vi "2013_01_05 Durability8 debug.vi"() -> ()   [LabVIEW 2012]
uses:
  MotorTypeDef.ctl
  <vilib>/DAQmx/write.llb/DAQmx Write (Counter Time 1Chan 1Samp).vi
  <vilib>/DAQmx/read.llb/DAQmx Read (Analog 1D Wfm NChan NSamp).vi
  <vilib>/Utility/TradDaqScaling.llb/Convert Thermistor Reading (waveform).vi
  <vilib>/DAQmx/miscellaneous.llb/DAQmx Fill In Error Info.vi
panel:
  out "XY Graph 2":cluster{"Array":dbl[], "Array":dbl[]}[](graph)
  out "Single Motor 2":waveform(dbl)[](graph)
  in  "Waveform":bool
  in  "Motor":dbl=1.0 min=1.0 max=8.0 step=1.0
  out "XY Graph":cluster{"Array":dbl[], "Array":dbl[]}(graph)
  out "error out":errorcluster
  in  "File Path":path=path "Durability/.lvm"
  in  "Motor 1":T1 {"Power Input (W)" format="%.3g"; "Efficiency" format="%#_3g%%"; "Power Output (W)" format="%.3g"; "Torque (mNm)" format="%.3g"; "Elapsed Time" format="%<%H:%M:%S>t"; "Supply (V)" format="%.2f"; "RPM" scale=0.0..40000.0 scale format="%#_4p"}
  out "Motor Temp":dbl(slide) scale=65.0..110.0
  out "Tank Temp":dbl(slide) scale=65.0..110.0
  in  "Temp Probe\nOn Motor":dbl=1.0
  out "loop time (ms)":u32
  in  "stop":bool
  in  "Unlock PWM":bool=TRUE
  in  "PWM 2":dbl(slide)=100.0 min=0.0 max=100.0 step=5.0 scale=0.0..100.0
  in  "PWM 1":dbl(slide) min=0.0 max=100.0 step=5.0 scale=0.0..100.0
  # "Enable"
  # "Fail"
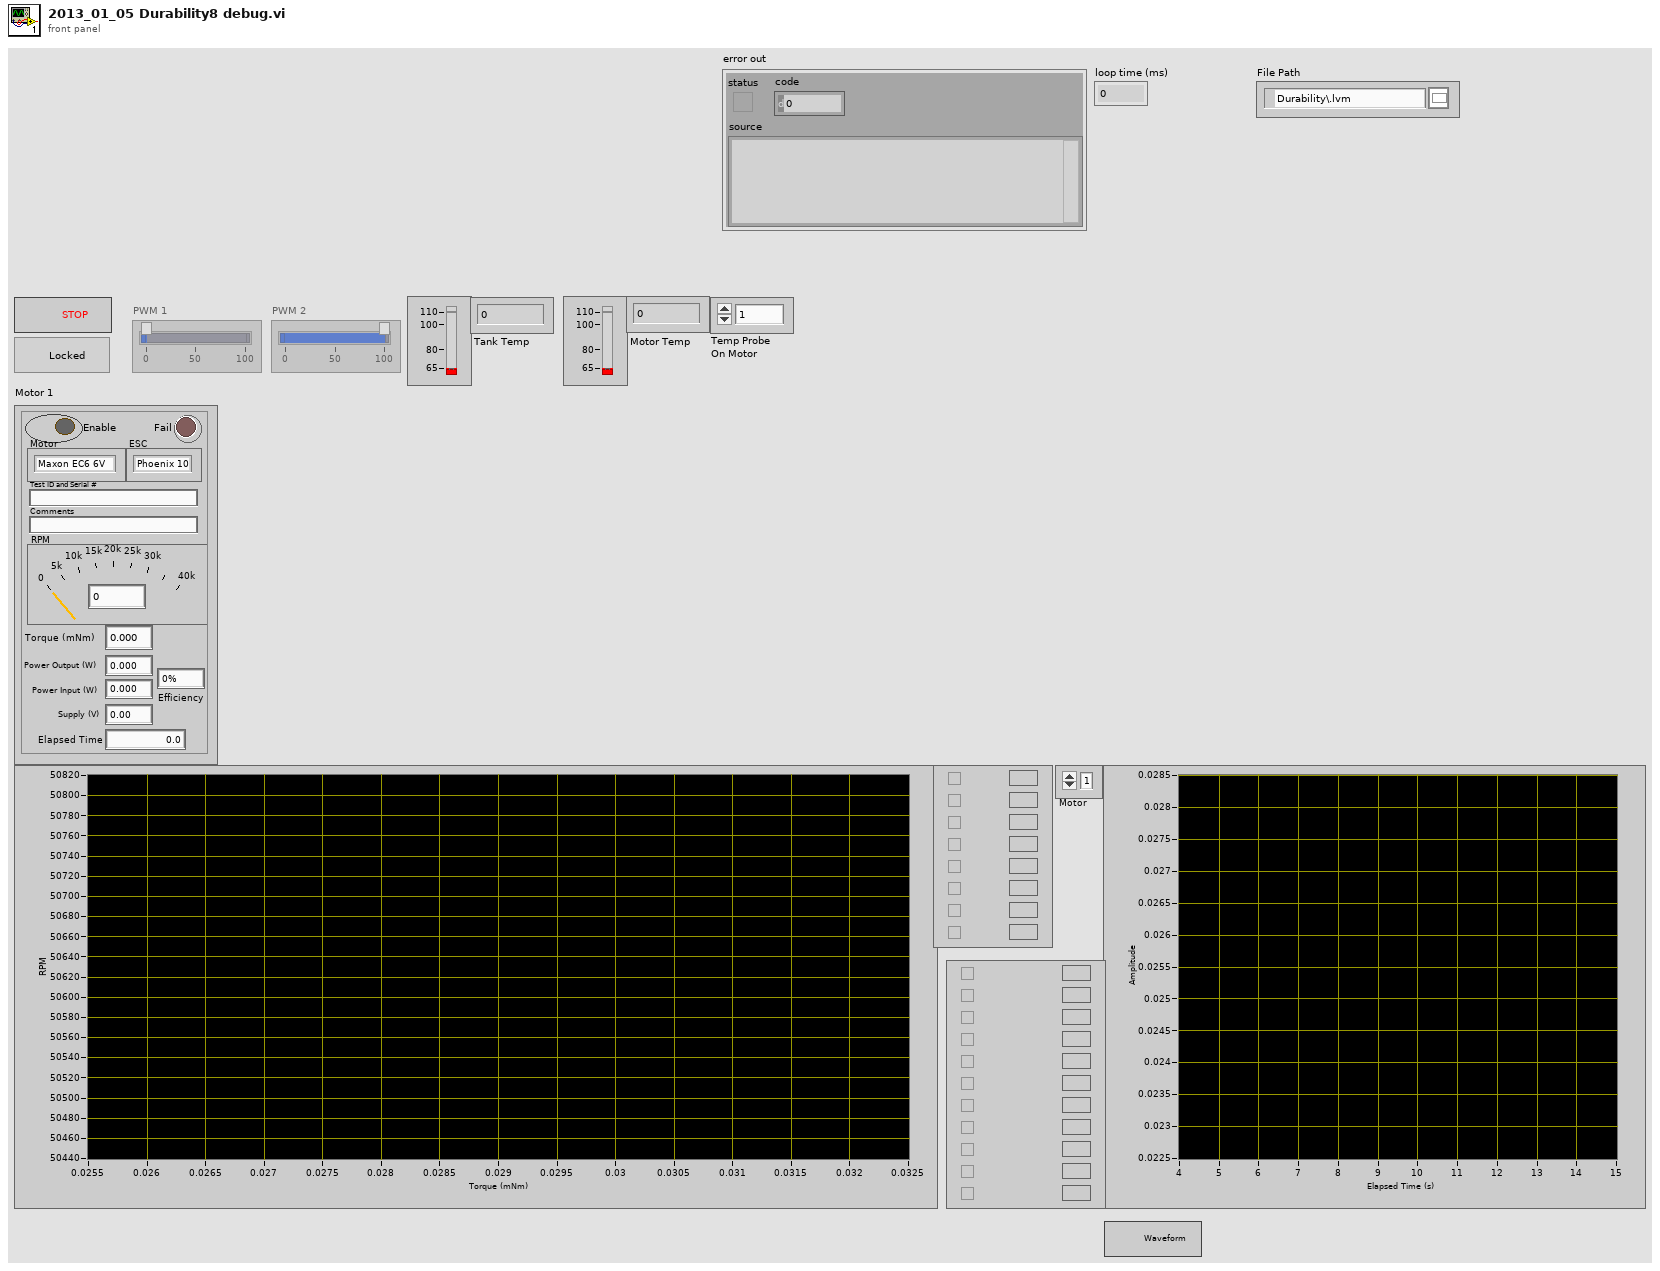
[diagram p1: front panel]
types:
  T1 = typedef "MotorTypeDef.ctl" = cluster{"Enabled":bool, "Fail":bool, "RPM":dbl, "Motor":enum16{"Maxon EC6 6V", "Maxon EC4 6V", "FH 0620 6V", "FH 0620 12V"}, "ESC":enum16{"Phoenix 10", "Maxon", "FH 1801"}, "Supply (V)":dbl, "Test ID and Serial #":string, "Comments":string, "Elapsed Time":dbl, "Counter":dbl, "Torque (mNm)":dbl, "Power Output (W)":dbl, "Efficiency":dbl, "Power Input (W)":dbl}
  T2 = enum8{"Enabled", "Disabled", "Disabled and Grayed Out"}
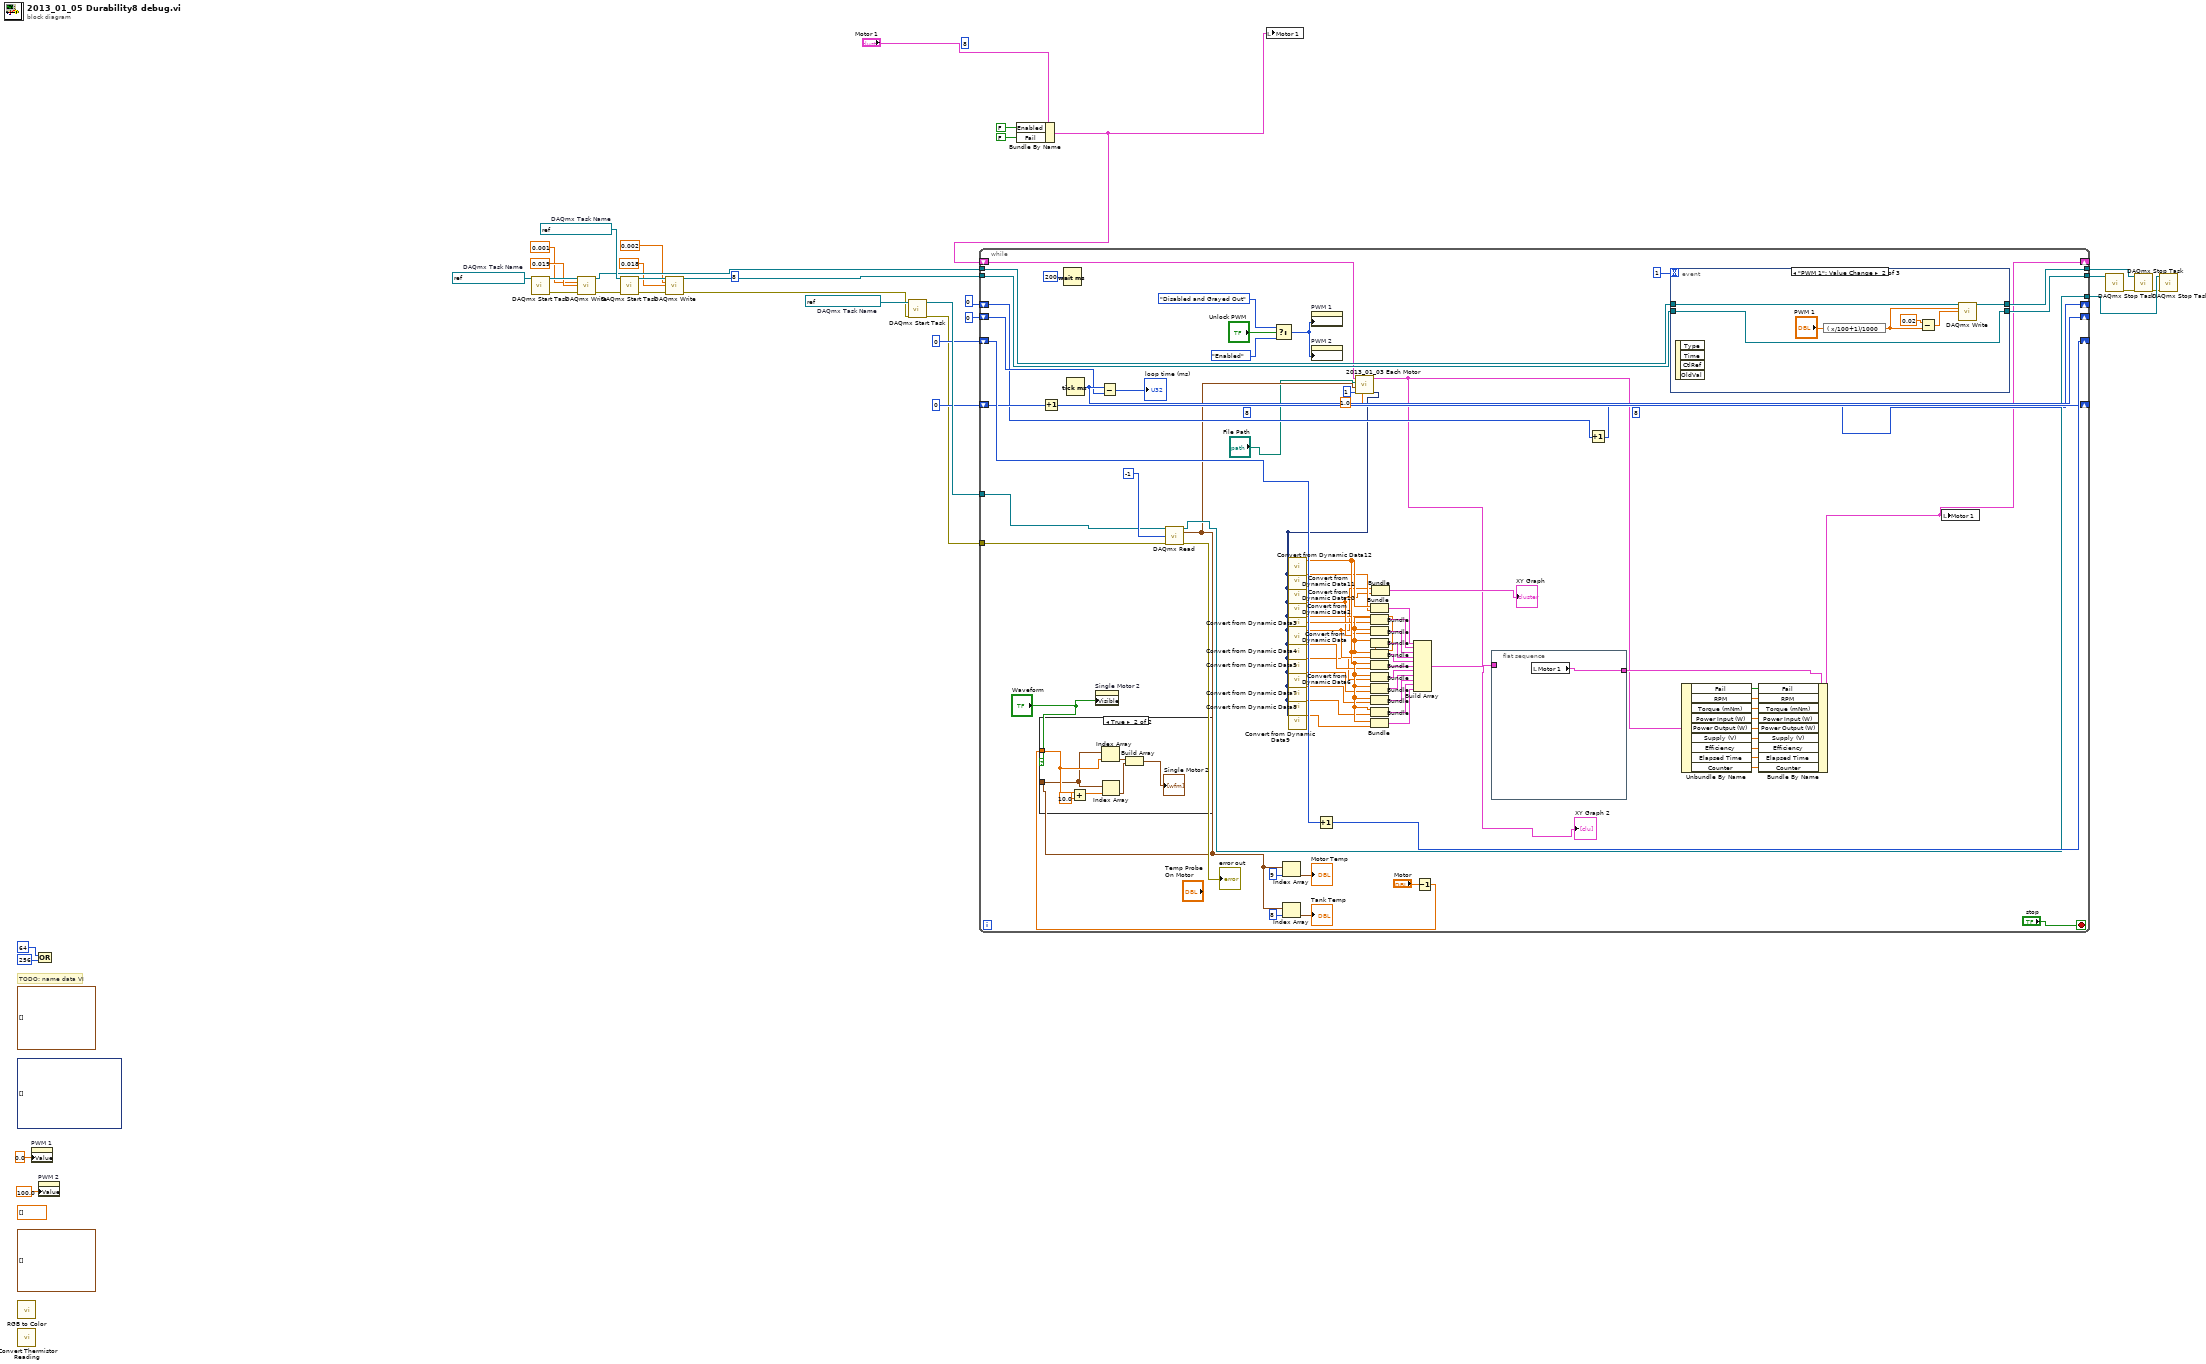
[diagram p0: block diagram]
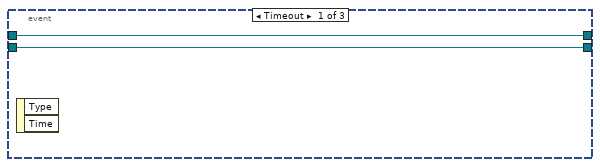
[diagram p3: hidden frame]
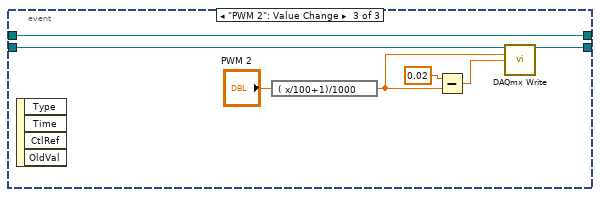
[diagram p4: hidden frame]
diagram:
  (unwired) 8
  (unwired) 8
  (unwired) dynamicdata[] []
  (unwired) dbl[] [] ("History Data")
  (unwired) waveform(dbl)[][] [] ("History Data")
  (unwired) waveform(dbl)[][] [] ("History Data")
  w30 = refnum<k21> "Durability8 PWM2"  # DAQmx Task Name
  w31 = refnum<k21> "Durability8 PWM1"  # DAQmx Task Name
  w34 = refnum<k21> "Durability8 Acquire"  # DAQmx Task Name
  # "TODO: name data VI"
  n1 = call <vilib>:"RGB to Color.vi"() -> ()  [unwired: 3 in, 1 out]
  n2 = call-poly <vilib>:"Convert Thermistor Reading.vi"() -> ()  [unwired: 7 in, 1 out]
  n3 = property on="PWM 1" class="Slide (strict)"("Value"=0.0 ("PWM 1")) -> ()  [unwired: 2 in, 2 out]
  n4 = Compound Arithmetic op=OR(64 ("options"), 256 ("options")) -> ()  [unwired: 1 out]
  n5 = property on="PWM 2" class="Slide (strict)"("Value"=100.0 ("PWM 2")) -> ()  [unwired: 2 in, 2 out]
  n6 = call <vilib>:"DAQmx Start Task.vi"("task/channels in"=w31) -> ("task out"=w27:refnum<k21>, "error out"=w25:errorcluster)  [unwired: 13 in]
  n7 = call-poly <vilib>:"DAQmx Write.vi"("task/channels in"=w27, "high time"=0.001 ("data"), "low time"=0.019 ("data"), "error in"=w25) -> ("task out"=w29:refnum<k21>, "error out"=w24:errorcluster)  [unwired: 9 in, 1 out]
  n8 = call <vilib>:"DAQmx Start Task.vi"("task/channels in"=w30, "error in"=w24) -> ("task out"=w26:refnum<k21>, "error out"=w23:errorcluster)  [unwired: 12 in]
  n9 = call-poly <vilib>:"DAQmx Write.vi"("task/channels in"=w26, "high time"=0.002 ("data"), "low time"=0.018 ("data"), "error in"=w23) -> ("task out"=w28:refnum<k21>, "error out"=w5:errorcluster)  [unwired: 9 in, 1 out]
  n10 = call <vilib>:"DAQmx Start Task.vi"("task/channels in"=w34, "error in"=w5) -> ("task out"=w33:refnum<k21>, "error out"=w6:errorcluster)  [unwired: 12 in]
  n11 = Bundle By Name(cluster="Motor 1", "Enabled"=FALSE, "Fail"=FALSE) -> (w1:T1)
  n12 = while {
    tunnel: w33 -> [w79]
    tunnel: [w80] -> w32
    tunnel: w6 -> [w92]
    shift-right: [w105] -> _
    shift-left: u32 0 ("millisecond timer value") -> [w104]
    tunnel: w29 -> [w97]
    tunnel: w28 -> [w96]
    tunnel: [w95] -> w22
    tunnel: [w94] -> w15
    shift-right: [w90] -> _
    shift-left: 0 ("for") -> [w91]
    shift-right: [w66] -> _
    shift-left: 0 ("for") -> [w67]
    shift-right: [w88] -> _
    shift-left: 0 ("for") -> [w89]
    shift-right: [w35] -> _
    shift-left: w1 -> [w78]
    stop <- "stop" stop-if-true
    (unwired) 8
    (unwired) 8
    n13 = Increment(x=w89) -> (x+1=w88:i32)
    n14 = Wait (ms)(milliseconds to wait=u32 200) -> ()  [unwired: 1 out]
    n15 = Tick Count (ms)() -> (millisecond timer value=w105:u32)
    n16 = property on="Single Motor 2" class="WFGraph (strict)"("Visible"="Waveform") -> ()  [unwired: 2 in, 2 out]
    n17 = Subtract(x=w105, y=w104) -> (x-y=→"loop time (ms)":u32)
    n18 = call-poly <vilib>:"DAQmx Read.vi"("task/channels in"=w79, "number of samples per channel"=-1, "error in"=w92) -> ("task out"=w80:refnum<k21>, "data"=w41:waveform(dbl)[], "error out"=→"error out":errorcluster)  [unwired: 10 in]
    n19 = Select(t=T2."Disabled and Grayed Out" ("Disabled"), s="Unlock PWM", f=T2."Enabled" ("Disabled")) -> (s? t:f=w109:T2)
    n20 = Index Array(array=w41, index=9) -> (element=→"Motor Temp":waveform(dbl))
    n21 = Index Array(array=w41, index=8) -> (element=→"Tank Temp":waveform(dbl))
    n22 = property on="PWM 1" class="Slide (strict)"("DisabledEnum"=w109) -> ()  [unwired: 2 in, 2 out]
    n23 = property on="PWM 2" class="Slide (strict)"("DisabledEnum"=w109) -> ()  [unwired: 2 in, 2 out]
    n24 = Increment(x=w91) -> (x+1=w90:i32)
    n25 = call "2013_01_03 Each Motor.vi"("Temp On"=1.0, "Motor #"=1, "data"=w41, "File Path"="File Path", "Motor Typedef"=w78) -> ("Final Out"=w38:dynamicdata, "Motor Typedef Out"=w36:T1)  [unwired: 5 in]
    n26 = call "Convert from Dynamic Data12"("Dynamic Data Type"=w38) -> ("Array"=w54:dbl[])  [unwired: 3 in]
    n27 = call "Convert from Dynamic Data11"("Dynamic Data Type"=w38) -> ("Array"=w53:dbl[])  [unwired: 3 in]
    n28 = call "Convert from Dynamic Data10"("Dynamic Data Type"=w38) -> ("Array"=w52:dbl[])  [unwired: 3 in]
    n29 = call "Convert from Dynamic Data2"("Dynamic Data Type"=w38) -> ("Array"=w51:dbl[])  [unwired: 3 in]
    n30 = call "Convert from Dynamic Data3"("Dynamic Data Type"=w38) -> ("Array"=w50:dbl[])  [unwired: 3 in]
    n31 = call "Convert from Dynamic Data"("Dynamic Data Type"=w38) -> ("Array"=w49:dbl[])  [unwired: 3 in]
    n32 = call "Convert from Dynamic Data4"("Dynamic Data Type"=w38) -> ("Array"=w48:dbl[])  [unwired: 3 in]
    n33 = call "Convert from Dynamic Data5"("Dynamic Data Type"=w38) -> ("Array"=w47:dbl[])  [unwired: 3 in]
    n34 = call "Convert from Dynamic Data6"("Dynamic Data Type"=w38) -> ("Array"=w46:dbl[])  [unwired: 3 in]
    n35 = call "Convert from Dynamic Data7"("Dynamic Data Type"=w38) -> ("Array"=w45:dbl[])  [unwired: 3 in]
    n36 = call "Convert from Dynamic Data8"("Dynamic Data Type"=w38) -> ("Array"=w44:dbl[])  [unwired: 3 in]
    n37 = call "Convert from Dynamic Data9"("Dynamic Data Type"=w38) -> ("Array"=w43:dbl[])  [unwired: 3 in]
    n38 = Bundle("Array"=w54, "Array"=w53) -> (w55:cluster{"Array":dbl[], "Array":dbl[]})  [unwired: 1 in]
    n39 = Bundle("Array"=w54, "Array"=w52) -> (w56:cluster{"Array":dbl[], "Array":dbl[]})  [unwired: 1 in]
    n40 = Bundle("Array"=w54, "Array"=w51) -> (w57:cluster{"Array":dbl[], "Array":dbl[]})  [unwired: 1 in]
    n41 = Bundle("Array"=w54, "Array"=w50) -> (w58:cluster{"Array":dbl[], "Array":dbl[]})  [unwired: 1 in]
    n42 = Bundle("Array"=w54, "Array"=w49) -> (w59:cluster{"Array":dbl[], "Array":dbl[]})  [unwired: 1 in]
    n43 = Bundle("Array"=w54, "Array"=w48) -> (w60:cluster{"Array":dbl[], "Array":dbl[]})  [unwired: 1 in]
    n44 = Bundle("Array"=w54, "Array"=w47) -> (w61:cluster{"Array":dbl[], "Array":dbl[]})  [unwired: 1 in]
    n45 = Bundle("Array"=w54, "Array"=w46) -> (w62:cluster{"Array":dbl[], "Array":dbl[]})  [unwired: 1 in]
    n46 = Bundle("Array"=w54, "Array"=w45) -> (w64:cluster{"Array":dbl[], "Array":dbl[]})  [unwired: 1 in]
    n47 = Bundle("Array"=w54, "Array"=w44) -> (w63:cluster{"Array":dbl[], "Array":dbl[]})  [unwired: 1 in]
    n48 = Bundle("Array"=w54, "Array"=w43) -> (w65:cluster{"Array":dbl[], "Array":dbl[]})  [unwired: 1 in]
    n49 = Bundle("Array"=w49, "Array"=w51) -> (→"XY Graph":cluster{"Array":dbl[], "Array":dbl[]})  [unwired: 1 in]
    n50 = Build Array(w55, w56, w57, w58, w59, w60, w61, w62, w64, w63, w65) -> (→"XY Graph 2":cluster{"Array":dbl[], "Array":dbl[]}[])
    n51 = Decrement(x="Motor") -> (x-1=w82:dbl)
    n52 = case shown="True" "Waveform" {
      tunnel: w41 -> [_ w114]
      tunnel: w82 -> [_ w115]
      frame False {
      }
      frame True {
        n53 = Add(x=w115, y=10.0) -> (x+y=w113:dbl)
        n54 = Index Array(array=w114, index=w115) -> (element=w112:waveform(dbl))
        n55 = Index Array(array=w114, index=w113) -> (element=w111:waveform(dbl))
        n56 = Build Array(w112, w111) -> (→"Single Motor 2":waveform(dbl)[])
      }
    }
    n57 = flat-sequence {
      tunnel: w36 -> [_]
      tunnel: [w117] -> w68
      frame #0 {
        n58 = local read "Motor 1"() -> (w117:T1)
      }
    }
    n59 = Increment(x=w67) -> (x+1=w66:i32)
    n60 = event shown="[1] \"PWM 1\": Value Change" {
      selector: _ -> [_ _ _]
      dyn-events: _ -> [_ _ _]
      timeout: 1 -> [_ _ _]
      tunnel: w97 -> [w119 w122 w128]
      tunnel: w96 -> [w118 w120 w127]
      tunnel: [w119 w121 w128] -> w95
      tunnel: [w118 w120 w129] -> w94
      event Timeout {
        n61 = event-data() -> ()  [unwired: 1 in, 2 out]
      }
      event "PWM 1": Value Change {
        n62 = event-data() -> ()  [unwired: 1 in, 4 out]
        n63 = expression code="( x/100+1)/1000"("PWM 1") -> (w123:dbl)
        n64 = Subtract(x=0.02 ("y"), y=w123) -> (x-y=w124:dbl)
        n65 = call-poly <vilib>:"DAQmx Write.vi"("task/channels in"=w122, "high time"=w123, "low time"=w124) -> ("task out"=w121:refnum<k21>)  [unwired: 10 in, 2 out]
      }
      event "PWM 2": Value Change {
        n66 = event-data() -> ()  [unwired: 1 in, 4 out]
        n67 = expression code="( x/100+1)/1000"("PWM 2") -> (w133:dbl)
        n68 = Subtract(x=0.02, y=w133) -> (x-y=w131:dbl)
        n69 = call-poly <vilib>:"DAQmx Write.vi"("task/channels in"=w127, "high time"=w133, "low time"=w131) -> ("task out"=w129:refnum<k21>)  [unwired: 10 in, 2 out]
      }
    }
    n70 = Unbundle By Name(w36) -> ("Fail"=w69:bool, "RPM"=w70:dbl, "Torque (mNm)"=w71:dbl, "Power Input (W)"=w72:dbl, "Power Output (W)"=w73:dbl, "Supply (V)"=w74:dbl, "Efficiency"=w75:dbl, "Elapsed Time"=w76:dbl, "Counter"=w77:dbl)
    n71 = Bundle By Name(cluster=w68, "Fail"=w69, "RPM"=w70, "Torque (mNm)"=w71, "Power Input (W)"=w72, "Power Output (W)"=w73, "Supply (V)"=w74, "Efficiency"=w75, "Elapsed Time"=w76, "Counter"=w77) -> (w35:T1)
    n72 = local write "Motor 1"(w35) -> ()
  }
  n73 = local write "Motor 1"(w1) -> ()
  n74 = call <vilib>:"DAQmx Stop Task.vi"("task/channels in"=w15) -> ("error out"=w21:errorcluster)  [unwired: 13 in, 1 out]
  n75 = call <vilib>:"DAQmx Stop Task.vi"("task/channels in"=w22, "error in"=w21) -> ("error out"=w20:errorcluster)  [unwired: 12 in, 1 out]
  n76 = call <vilib>:"DAQmx Stop Task.vi"("task/channels in"=w32, "error in"=w20) -> ()  [unwired: 12 in, 2 out]
